vi "Trim Project File Extension.vi"(8 "Error In":errorcluster, 11 "Project File Name":string) -> (0 "Error Out":errorcluster, 3 "Project Name":string)   [LabVIEW 2017, in "Bookmark Manager.lvlib"]
uses:
  Bookmark Manager.lvlib
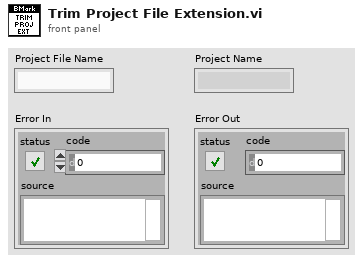
[diagram p1: front panel]
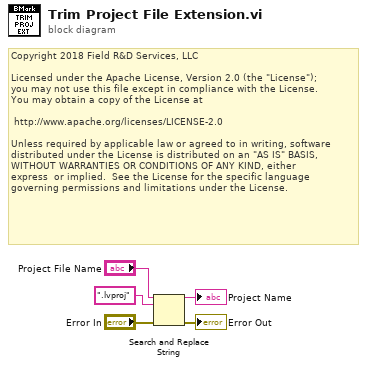
[diagram p0: block diagram]
diagram:
  # "Copyright 2018 Field R&D Services, LLC\n\nLicensed under the Apache License, Version 2.0 (the \"License\");\nyou may not use this file except in compliance with the License.\nYou may obtain a copy of the License at\n\n\thttp://www.apache.org/licenses/LICENSE-2.0\n\nUnless required by applicable law or agreed to in writing, software\ndistributed under the License is distributed on an \"AS IS\" BASIS,\nWITHOUT WARRANTIES OR CONDITIONS OF ANY KIND, either \nexpress  or implied.  See the License for the specific language \ngoverning permissions and limitations under the License."
  n1 = Search and Replace String(input string="Project File Name", search string=".lvproj", error in="Error In") -> (result string=→"Project Name":string, error out=→"Error Out":errorcluster)  [unwired: 5 in, 2 out]
